vi "BRig_Host_v0,53.vi"() -> ()   [LabVIEW 2014]
uses:
  <vilib>/WebDAVClient/Advanced/SessionHandle.ctl
  BRig_Host__global__stopHost.vi
  <vilib>/Utility/file.llb/Write To Spreadsheet File (DBL).vi
  <vilib>/WebDAVClient/NI_WebDAV.lvlib
panel:
  out "FreeReward_c_R":u16
  out "FreeReward_c_L":u16
  out "BTPR_avg_R":dbl
  out "T2R_avg_R":dbl
  out "BTPR_avg_L":dbl
  out "T2R_avg_L":dbl
  out "BTPR_cur":u16
  out "T2R_cur":u16
  out "nReward":u16 caption="# Rewards in Current Block"
  out "BUR_target":u16 caption="Target Trials Per Block"
  out "nTrial":u16
  out "nReward_Right":u16 caption="# Rewards Total (Right)"
  out "nReward_Left":u16 caption="# Rewards Total (Left)"
  out "nReward_cur":u16 caption="# Rewards in Current Block"
  out "TpB_target":u16 caption="Target Trials Per Block"
  out "iBlock":u16 caption="Current Block"
  out "iTrial":u16 caption="Current Trial"
  out "DAB_nRewards_ProbLow_percent":u16 caption="# Rewards Total (Right)"
  out "DAB_nRewards_ProbHigh_percent":u16 caption="# Rewards Total (Left)"
  out "DAB_nRewards_ProbLow":u16 caption="# Rewards Total (Right)"
  out "DAB_nRewards_ProbHigh":u16 caption="# Rewards Total (Left)"
  out "DAB_nRewards_total":u16 caption="# Rewards in Current Block"
  out "DAB_nTrial":u16
  out "DAB_nRewards_Right":u16 caption="# Rewards Total (Right)"
  out "DAB_nRewards_Left":u16 caption="# Rewards Total (Left)"
  out "writeError":bool
  out "error IO":errorcluster
  out "error_loopP_loadSettings":errorcluster caption="error out"
  out "testCmdList":u16[][](array[numeric])
  in  "ClosedLoop":bool
  in  "module":string=" module1 "
  in  "input_updateTrial_subsequent":u16
  in  "input_updateTrial_first":u16
  in  "input_forceUpdate":bool
  in  "ClosedLoop":u16[](array[numeric])
  in  "testNewLaserSettings":bool
  in  "LoadSettings":bool
  in  "DisplayNumber":u16
  out "XY Graph":cluster{u16[], u16[]}[](graph)
  in  "threshold_2":u16=600
  in  "threshold_1":u16=300
  in  "Port (F=A/B, T=C)":bool
  out "I_ExpRun":bool
  out "TCP_connection":bool
  in  "stopHost":bool
  # "# Trials Displayed\n( 0 = all )"
  # "Selection\nTime Thresholds"
  # "Dual Armed Bandit"
  # "Standard or 2 Cues"
  # "Total"
  # "# Rewards"
  # "# Trials"
  # "Block Target"
  # "# Blocks"
  # "# Trials"
  # "# Rewards"
  # "Left           Right"
  # "Bad Trials\nPost Reward"
  # "Trials 2 Reward"
  # "Block"
  # "# Selections"
  # "# Trials"
  # "# Rewards"
  # "Current\nBlock"
  # "High Prob    Low Prob"
  # "avg L"
  # "Total"
  # "# Rewards"
  # "# Trials"
  # "avg R"
  # "% Selections"
  # "High Prob    Low Prob"
  # "FreeRewards"
  # "Left           Right"
  # "Port Switch\nToggle TRUE if debugging"
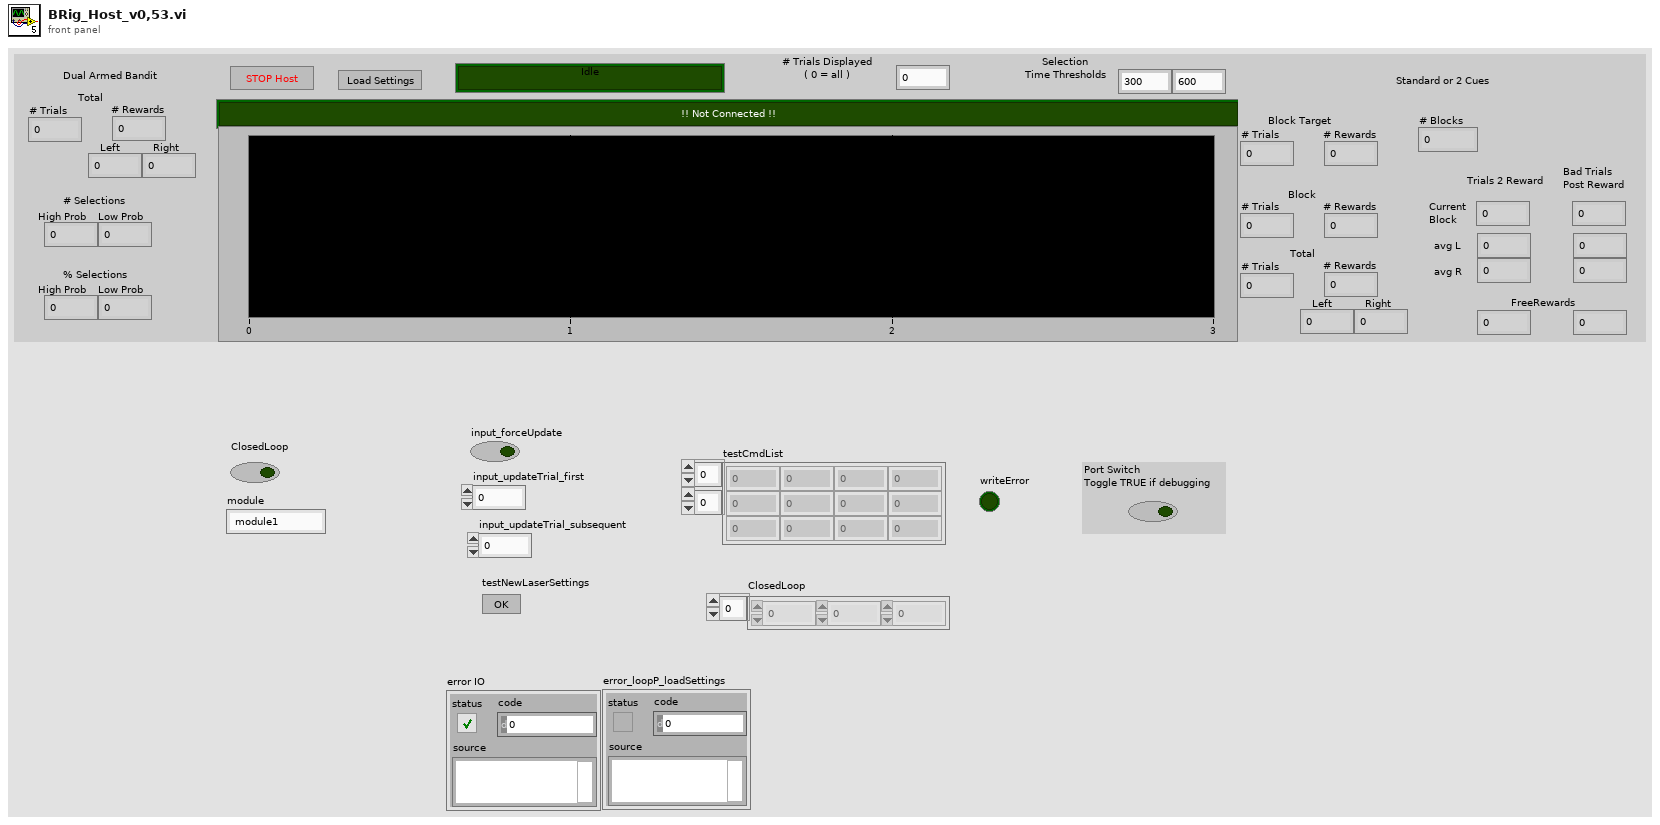
[diagram p1: front panel]
types:
  T1 = typedef "NI_WebDAV.lvlib/SessionHandle.ctl" = refnum<k1>
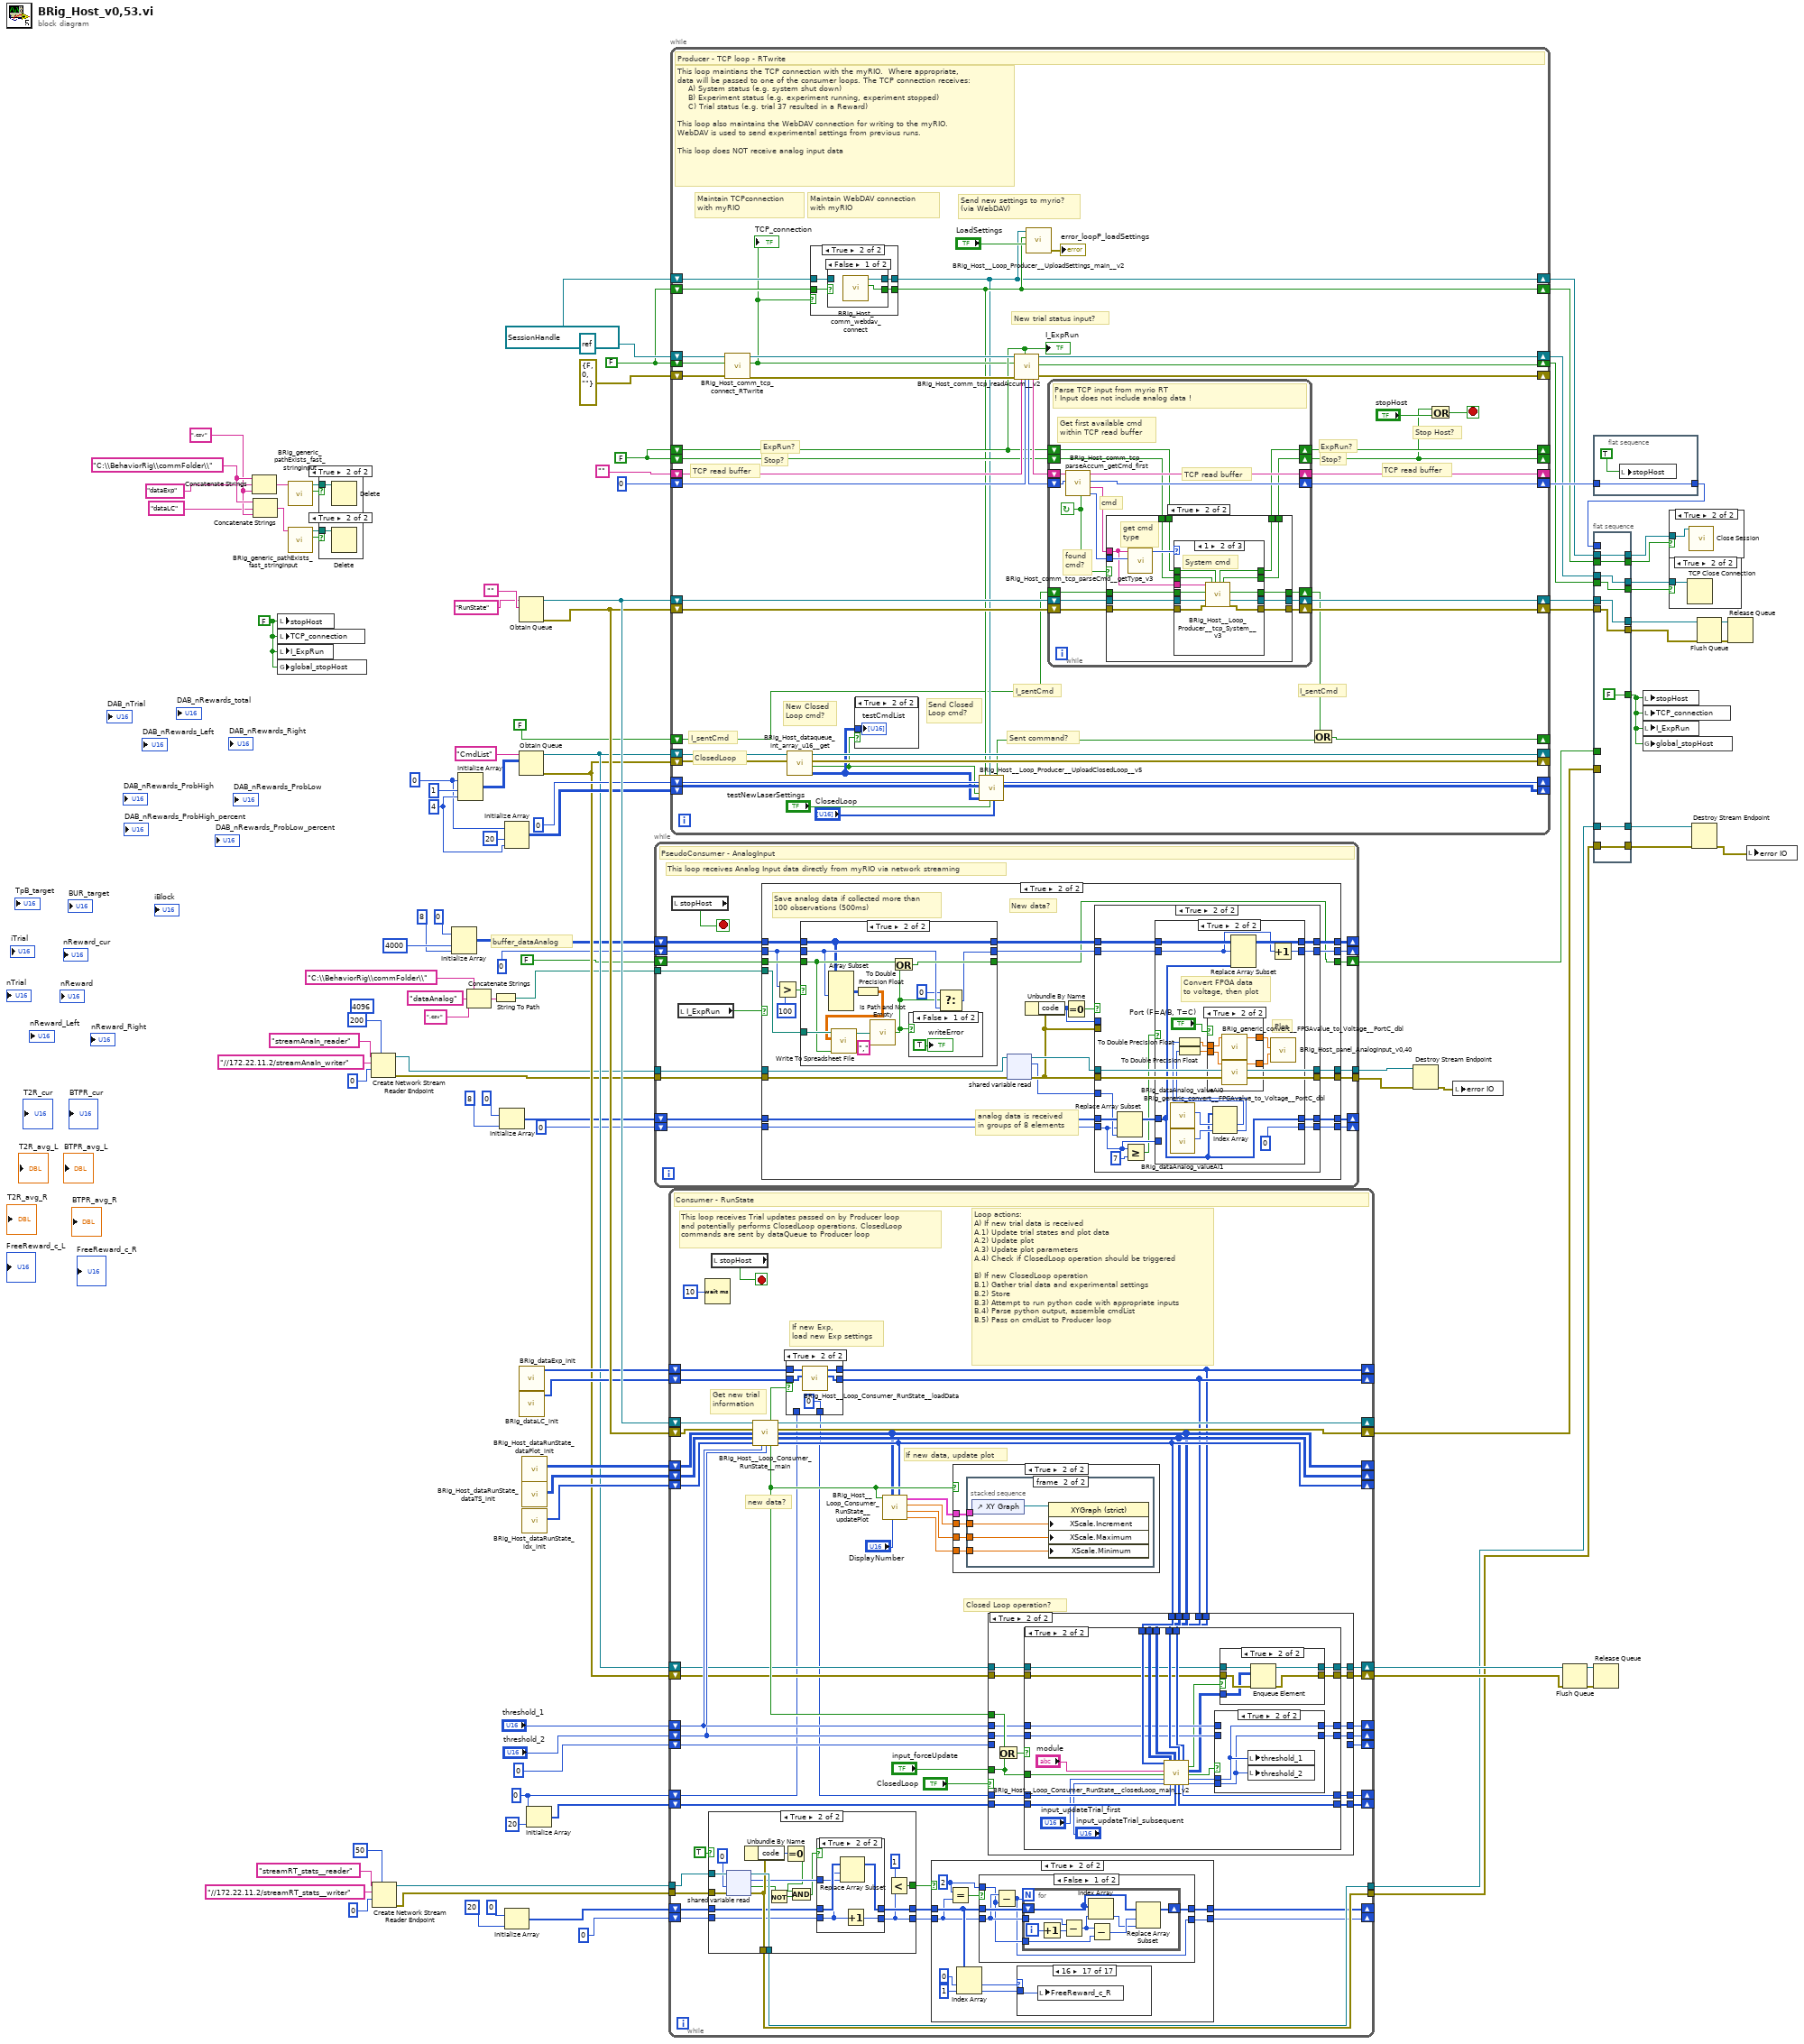
[diagram p0: block diagram]
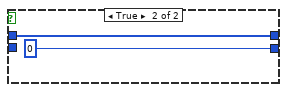
[diagram p9: hidden frame]
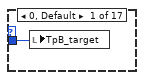
[diagram p10: hidden frame]
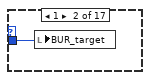
[diagram p11: hidden frame]
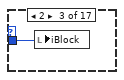
[diagram p12: hidden frame]
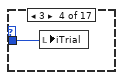
[diagram p13: hidden frame]
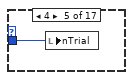
[diagram p14: hidden frame]
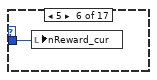
[diagram p15: hidden frame]
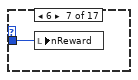
[diagram p16: hidden frame]
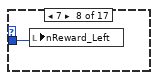
[diagram p17: hidden frame]
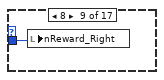
[diagram p18: hidden frame]
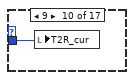
[diagram p19: hidden frame]
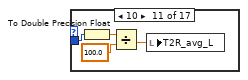
[diagram p20: hidden frame]
diagram:
  (unwired) 4096 ("reader buffer size")
  w41 = u16 0 ("element")
  w42 = 4 ("dimension size")
  w58 = u16 0
  w70 = ".csv" ("string")
  w71 = "C:\\BehaviorRig\\commFolder\\"
  w83 = T1 refnum items=["Session NI_WebDAV"] ("session handle")
  w101 = FALSE ("stopHost")
  w102 = FALSE
  w84 = FALSE
  # "buffer_dataAnalog"
  n1 = Concatenate Strings(w71, "dataExp" ("string"), w70) -> (w65:string)
  n2 = Concatenate Strings(w71, "dataLC" ("string"), w70) -> (w62:string)
  n3 = local write "stopHost"(w101) -> ()
  n4 = local write "TCP_connection"(w101) -> ()
  n5 = local write "I_ExpRun"(w101) -> ()
  n6 = global write "BRig_Host__global__stopHost.vi" "global_stopHost"(w101) -> ()
  n7 = call "BRig_generic_pathExists_fast_stringInput.vi"("input_filePath"=w65) -> ("output_Iexist"=w67:bool, "output_filePath"=w66:path)  [unwired: 8 in, 1 out]
  n8 = call "BRig_generic_pathExists_fast_stringInput.vi"("input_filePath"=w62) -> ("output_Iexist"=w63:bool, "output_filePath"=w64:path)  [unwired: 8 in, 1 out]
  n9 = case shown="True" w67 {
    tunnel: w66 -> [_ w107]
    frame False {
    }
    frame True {
      n10 = Delete(path (use dialog)=w107) -> ()  [unwired: 4 in, 3 out]
    }
  }
  n11 = case shown="True" w63 {
    tunnel: w64 -> [_ w108]
    frame False {
    }
    frame True {
      n12 = Delete(path (use dialog)=w108) -> ()  [unwired: 4 in, 3 out]
    }
  }
  n13 = Create Network Stream Reader Endpoint(7:200 ("reader buffer size"), 9:u16 0 ("element"), 10:"//172.22.11.2/streamAnaIn_writer" ("writer url"), 11:"streamAnaIn_reader" ("reader name")) -> (0:w25:errorcluster, 3:w26:refnum<k21>)  [unwired: 3 in]
  n14 = Create Network Stream Reader Endpoint(7:50 ("reader buffer size"), 9:u16 0 ("element"), 10:"//172.22.11.2/streamRT_stats__writer" ("writer url"), 11:"streamRT_stats__reader" ("reader name")) -> (0:w11:errorcluster, 3:w12:refnum<k21>)  [unwired: 3 in]
  n15 = Initialize Array(u16 0 ("element"), 4000 ("dimension size"), 8 ("dimension size")) -> (w37:u16[][])
  n16 = Initialize Array(w41, 1 ("dimension size"), w42) -> (w53:u16[][])
  n17 = Concatenate Strings("C:\\BehaviorRig\\commFolder\\" ("string"), "dataAnalog" ("input_filename"), ".csv" ("string")) -> (w34:string)
  n18 = String To Path(string=w34) -> (path=w31:path)
  n19 = Initialize Array(u16 0 ("element"), 8 ("dimension size")) -> (w18:u16[])
  n20 = Initialize Array(w41, 20 ("dimension size"), w42) -> (w72:u16[][])
  n21 = Initialize Array(u16 0 ("element"), 20 ("dimension size")) -> (w8:u16[])
  n22 = Obtain Queue(name (unnamed)="RunState", element data type="") -> (queue out=w93:refnum<queue>, error out=w92:errorcluster)  [unwired: 3 in, 1 out]
  n23 = Obtain Queue(name (unnamed)="CmdList", element data type=w53) -> (queue out=w52:refnum<queue>, error out=w51:errorcluster)  [unwired: 3 in, 1 out]
  n24 = call "BRig_dataExp_init.vi"() -> ("output_dataExp"=w61:u16[])  [unwired: 11 in]
  n25 = call "BRig_dataLC_init.vi"() -> ("output_dataLC"=w60:u16[])  [unwired: 11 in]
  n26 = call "BRig_Host_dataRunState_dataPlot_init.vi"() -> ("output_dataPlot"=w89:u16[][])  [unwired: 11 in]
  n27 = call "BRig_Host_dataRunState_dataTS_init.vi"() -> ("output_dataTS"=w88:u16[][])  [unwired: 11 in]
  n28 = call "BRig_Host_dataRunState_idx_init.vi"() -> ("output_idx"=w87:i32[])  [unwired: 11 in]
  n29 = Initialize Array(w58, 20 ("dimension size")) -> (w56:u16[])
  n30 = while {
    shift-right: [w123] -> _
    shift-left: w37 -> [w125]
    shift-right: [w122] -> _
    shift-left: 0 -> [w124]
    tunnel: w31 -> [w121]
    shift-right: [w119] -> w29
    shift-left: FALSE -> [w120]
    tunnel: w26 -> [w117]
    tunnel: w25 -> [w116]
    tunnel: [w115] -> w23
    tunnel: [w114] -> w22
    shift-right: [w111] -> _
    shift-left: w18 -> [w113]
    shift-right: [w110] -> _
    shift-left: 0 ("element") -> [w112]
    stop <- w109 stop-if-true
    # "This loop receives Analog Input data directly from myRIO via network streaming"
    # "PseudoConsumer - AnalogInput"
    n31 = local read "stopHost"() -> (w109:bool)
    n32 = local read "I_ExpRun"() -> (w118:bool)
    n33 = case shown="True" w118 {
      tunnel: w125 -> [w132 w156]
      tunnel: w124 -> [_ w142]
      tunnel: [w132 w151] -> w123
      tunnel: [0 w149] -> w122
      tunnel: w121 -> [_ w154]
      tunnel: w120 -> [_ w155]
      tunnel: [FALSE w139] -> w119
      tunnel: w117 -> [w129 w148]
      tunnel: w116 -> [w128 w147]
      tunnel: [w129 w145] -> w115
      tunnel: [w128 w143] -> w114
      tunnel: w113 -> [w127 w137]
      tunnel: w112 -> [_ w136]
      tunnel: [w127 w135] -> w111
      tunnel: [0 ("element") w134] -> w110
      frame False {
        n34 = Wait (ms)(milliseconds to wait=u32 20) -> ()  [unwired: 1 out]
      }
      frame True {
        # "analog data is received\nin groups of 8 elements"
        # "New data?"
        # "Save analog data if collected more than\n100 observations (500ms)"
        n35 = Greater?(x=w142, y=100) -> (0:w157:bool)
        n36 = case shown="True" w157 {
          tunnel: w156 -> [w216 w219]
          tunnel: [w216 w219] -> w152
          tunnel: w142 -> [w215 w221]
          tunnel: w155 -> [w214 w223]
          tunnel: [w215 w220] -> w150
          tunnel: [w214 w222] -> w139
          tunnel: w154 -> [_ w228]
          frame False {
          }
          frame True {
            n37 = Array Subset(array=w219, length (row)=w221) -> (w227:u16[][])  [unwired: 3 in]
            n38 = To Double Precision Float(number=w227) -> (double precision float=w226:dbl[][])
            n39 = call-poly <vilib>:"Write To Spreadsheet File.vi"("delimiter (\\t)"="," ("delimiter (\\t)"), "append to file? (new file:F)"=w223, "2D data"=w226, "file path (dialog if empty)"=w228) -> ("new file path (Not A Path if cancelled)"=w224:path)  [unwired: 4 in]
            n40 = call <vilib>:"Is Path and Not Empty.vi"("path"=w224) -> ("Is Path and Not Empty?"=w217:bool)  [unwired: 4 in]
            n41 = Or(x=w223, y=w217) -> (x .or. y?=w222:bool)
            n42 = case shown="False" w217 {
              frame False {
                "writeError" <- TRUE ("writeError")
              }
              frame True {
              }
            }
            n43 = Select(t=0, s=w217, f=w221) -> (s? t:f=w220:i32)
          }
        }
        n44 = shared-variable-read(w148, w147) -> (w146:refnum<k21>, w144:errorcluster, w138:u16)  [unwired: 1 in, 1 out]
        n45 = Unbundle By Name(w144) -> ("code"=w140:i32)
        n46 = Equal To 0?(x=w140) -> (x = 0?=w153:bool)
        n47 = case shown="True" w153 {
          tunnel: w152 -> [w170 w185]
          tunnel: [w170 w184] -> w151
          tunnel: w150 -> [w169 w183]
          tunnel: [w169 w182] -> w149
          tunnel: w144 -> [w167 _]
          tunnel: w146 -> [w166 w181]
          tunnel: [w166 w181] -> w145
          tunnel: w144 -> [w165 w180]
          tunnel: [w165 w180] -> w143
          tunnel: w140 -> [w164 _]
          tunnel: w138 -> [_ w178]
          tunnel: w137 -> [w159 w179]
          tunnel: w136 -> [w158 w176]
          tunnel: [w159 w173] -> w135
          tunnel: [w158 w175] -> w134
          frame False {
            n48 = Equal?(x=-314100, y=w164) -> (x = y?=w162:bool)
            n49 = Equal?(x=-314220, y=w164) -> (x = y?=w161:bool)
            n50 = Or(x=w162, y=w161) -> (x .or. y?=w160:bool)
            n51 = case shown="False" w160 {
              tunnel: w167 -> [w171 _]
              frame False {
                "error IO" <- w171
              }
              frame True {
              }
            }
          }
          frame True {
            n52 = Replace Array Subset(array=w179, new element=w178, index=w176) -> (w174:u16[])
            n53 = Greater Or Equal?(x=w176, y=7) -> (x >= y?=w172:bool)
            n54 = case shown="True" w172 {
              tunnel: w185 -> [w190 w205]
              tunnel: [w190 w204] -> w184
              tunnel: w183 -> [w189 w203]
              tunnel: [w189 w202] -> w182
              tunnel: w176 -> [w188 _]
              tunnel: [w187 0 ("y")] -> w175
              tunnel: w174 -> [w186 w193]
              tunnel: [w186 w193] -> w173
              frame False {
                n55 = Increment(x=w188) -> (x+1=w187:i32)
              }
              frame True {
                # "Convert FPGA data\nto voltage, then plot"
                # "Plot"
                n56 = call "BRig_dataAnalog_valueAI0.vi"() -> ("output_valueAI0"=w195:i32)  [unwired: 11 in]
                n57 = call "BRig_dataAnalog_valueAI1.vi"() -> ("output_valueAI1"=w196:i32)  [unwired: 11 in]
                n58 = Index Array(array=w193, index #1=w195, index #2=w196) -> (element #1=w192:u16, element #2=w191:u16)
                n59 = To Double Precision Float(number=w192) -> (double precision float=w197:dbl)
                n60 = To Double Precision Float(number=w191) -> (double precision float=w198:dbl)
                n61 = case shown="True" "Port (F=A/B, T=C)" {
                  tunnel: w197 -> [w207 w213]
                  tunnel: w198 -> [w206 w212]
                  tunnel: [w209 w211] -> w200
                  tunnel: [w208 w210] -> w199
                  frame False {
                    n62 = call "BRig_generic_convert__FPGAvalue_to_Voltage__PortAorB_dbl.vi"("input_FPGAvalue_PortAorB"=w207) -> ("output_voltage"=w209:dbl)  [unwired: 10 in]
                    n63 = call "BRig_generic_convert__FPGAvalue_to_Voltage__PortAorB_dbl.vi"("input_FPGAvalue_PortAorB"=w206) -> ("output_voltage"=w208:dbl)  [unwired: 10 in]
                  }
                  frame True {
                    n64 = call "BRig_generic_convert__FPGAvalue_to_Voltage__PortC_dbl.vi"("input_FPGAvalue_PortC"=w213) -> ("output_voltage"=w211:dbl)  [unwired: 10 in]
                    n65 = call "BRig_generic_convert__FPGAvalue_to_Voltage__PortC_dbl.vi"("input_FPGAvalue_PortC"=w212) -> ("output_voltage"=w210:dbl)  [unwired: 10 in]
                  }
                }
                n66 = Replace Array Subset(array=w205, new element=w193, index (row)=w203) -> (w204:u16[][])  [unwired: 1 in]
                n67 = Increment(x=w203) -> (x+1=w202:i32)
                n68 = call "BRig_Host_panel_AnalogInput_v0,40.vi"("graph_ai1"=w199, "graph_ai0"=w200) -> ()  [unwired: 10 in]
              }
            }
          }
        }
      }
    }
  }
  n69 = while {
    shift-right: [w274] -> _
    shift-left: w93 -> [w275]
    shift-right: [w272] -> w46
    shift-left: w92 -> [w273]
    shift-right: [w255] -> _
    shift-left: w89 -> [w271]
    shift-right: [w256] -> _
    shift-left: w88 -> [w270]
    shift-right: [w257] -> _
    shift-left: w87 -> [w269]
    shift-right: [w265] -> _
    shift-left: "threshold_1" -> [w264]
    shift-right: [w263] -> _
    shift-left: "threshold_2" -> [w262]
    shift-right: [w253] -> _
    shift-left: w61 -> [w267]
    shift-right: [w254] -> _
    shift-left: w60 -> [w266]
    shift-right: [w247] -> _
    shift-left: w58 -> [w245]
    shift-right: [w259] -> _
    shift-left: u8 0 -> [w260]
    shift-right: [w246] -> _
    shift-left: w56 -> [w243]
    shift-right: [w250] -> w48
    shift-left: w52 -> [w252]
    shift-right: [w249] -> w47
    shift-left: w51 -> [w251]
    tunnel: w12 -> [w241]
    tunnel: w11 -> [w240]
    shift-right: [w232] -> _
    shift-left: w8 -> [w237]
    shift-right: [w231] -> _
    shift-left: 0 ("element") -> [w236]
    tunnel: [w239] -> w4
    tunnel: [w238] -> w3
    stop <- w242 stop-if-true
    # "Closed Loop operation?"
    # "Loop actions:\nA) If new trial data is received\nA.1) Update trial states and plot data\nA.2) Update plot\nA.3) Update plot parameters\nA.4) Check if ClosedLoop operation should be triggered\n\nB) If new ClosedLoop operation\nB.1) Gather trial data and experimental settings\nB.2) Store\nB.3) Attempt to run python code with appropriate inputs\nB.4) Parse python output, assemble cmdList\nB.5) Pass on cmdList to Producer loop"
    # "This loop receives Trial updates passed on by Producer loop\nand potentially performs ClosedLoop operations. ClosedLoop\ncommands are sent by dataQueue to Producer loop"
    # "If new data, update plot"
    # "If new Exp,\nload new Exp settings"
    # "new data?"
    # "Get new trial\ninformation"
    # "Consumer - RunState"
    n70 = Wait (ms)(milliseconds to wait=u32 10) -> ()  [unwired: 1 out]
    n71 = case shown="True" TRUE {
      selector: TRUE -> [w282 _]
      tunnel: w241 -> [w286 w302]
      tunnel: w240 -> [w285 w301]
      tunnel: [w286 w300] -> w239
      tunnel: [w285 w299] -> w238
      tunnel: w237 -> [w284 w297]
      tunnel: w236 -> [w283 w296]
      tunnel: [w282 w294] -> w235
      tunnel: [w284 w293] -> w234
      tunnel: [w283 w292] -> w233
      frame False {
      }
      frame True {
        n72 = shared-variable-read(w302, w301, 0 ("timeout ms (-1)")) -> (w300:refnum<k21>, w299:errorcluster, w290:bool, w298:u16)
        n73 = Unbundle By Name(w299) -> ("code"=w303:i32)
        n74 = Not(x=w290) -> (.not. x?=w289:bool)
        n75 = Equal To 0?(x=w303) -> (x = 0?=w288:bool)
        n76 = And(x=w288, y=w289) -> (x .and. y?=w287:bool)
        n77 = case shown="True" w287 {
          tunnel: w298 -> [_ w309]
          tunnel: w297 -> [w305 w310]
          tunnel: w296 -> [w304 w308]
          tunnel: [w305 w306] -> w293
          tunnel: [w304 w307] -> w292
          frame False {
          }
          frame True {
            n78 = Replace Array Subset(array=w310, new element=w309, index=w308) -> (w306:u16[])
            n79 = Increment(x=w308) -> (x+1=w307:i32)
          }
        }
        n80 = Less?(x=1, y=w292) -> (x < y?=w294:bool)
      }
    }
    n81 = local read "stopHost"() -> (w242:bool)
    n82 = call "BRig_Host__Loop_Consumer_RunState__main.vi"("input_hDataQueue"=w275, "input_errorDataQueue"=w273, "input_dataPlot"=w271, "input_dataTS"=w270, "input_idx"=w269, "threshold_1"=w264, "threshold_2"=w262) -> ("output_ExpStart"=w268:bool, "output_hDataQueue"=w274:refnum<queue>, "output_errorDataQueue"=w272:errorcluster, "output_dataPlot"=w255:u16[][], "output_dataTS"=w256:u16[][], "output_updatePlot"=w258:bool, "output_idx"=w257:i32[])  [unwired: 2 in]
    n83 = case shown="True" w268 {
      tunnel: w267 -> [w451 w453]
      tunnel: [w451 w456] -> w253
      tunnel: w266 -> [w450 w454]
      tunnel: [w450 w455] -> w254
      tunnel: w245 -> [w449 _]
      tunnel: [w449 u16 0] -> w244
      frame False {
      }
      frame True {
        n84 = call "BRig_Host__Loop_Consumer_RunState__loadData.vi"("input_dataLC"=w454, "input_dataExp"=w453) -> ("output_dataLC"=w455:u16[], "output_dataExp"=w456:u16[])  [unwired: 8 in]
      }
    }
    n85 = call "BRig_Host__Loop_Consumer_RunState__updatePlot.vi"("input_idx"=w257, "input_DisplayNumber"="DisplayNumber", "input_dataPlot"=w255, "input_updatePlot"=w258) -> ("output_X_min"=w278:dbl, "output_X_max"=w277:dbl, "output_X_inc"=w276:dbl, "XY Graph"=w279:cluster{u16[], u16[]}[])  [unwired: 4 in]
    n86 = case shown="True" w235 {
      tunnel: w234 -> [w312 w317]
      tunnel: w233 -> [w311 w315]
      tunnel: [w312 w316] -> w232
      tunnel: [w311 w314] -> w231
      frame False {
      }
      frame True {
        w313 = 2 ("x")
        n87 = Equal?(x=w313, y=w315) -> (x = y?=w318:bool)
        n88 = Index Array(array=w317, index #1=0 ("index"), index #2=1 ("index")) -> (element #1=w320:u16, element #2=w319:u16)
        n89 = case shown="False" w318 {
          tunnel: w317 -> [w327 w338]
          tunnel: [w323 w338] -> w316
          tunnel: w315 -> [w326 _]
          tunnel: [w324 0 ("index")] -> w314
          tunnel: w313 -> [w325 _]
          frame False {
            n90 = Subtract(x=w326, y=w325) -> (x-y=w324:i32)
            n91 = for {
              N: w324 -> [_]
              shift-right: [w328] -> w323
              shift-left: w327 -> [w331]
              tunnel: w326 -> [w334]
              tunnel: w325 -> [w333]
              i -> [w336]
              n92 = Increment(x=w336) -> (x+1=w335:i32)
              n93 = Subtract(x=w334, y=w335) -> (x-y=w332:i32)
              n94 = Index Array(array=w331, index=w332) -> (element=w329:u16)
              n95 = Subtract(x=w332, y=w333) -> (x-y=w330:i32)
              n96 = Replace Array Subset(array=w331, new element=w329, index=w330) -> (w328:u16[])
            }
          }
          frame True {
          }
        }
        n97 = case shown="16" w320 {
          tunnel: w319 -> [w339 w340 w341 w342 w343 w344 w345 w346 w347 w348 w352 w356 w357 w359 w363 w366 w367]
          frame 0, Default {
            n98 = local write "TpB_target"(w339) -> ()
          }
          frame 1 {
            n99 = local write "BUR_target"(w340) -> ()
          }
          frame 2 {
            n100 = local write "iBlock"(w341) -> ()
          }
          frame 3 {
            n101 = local write "iTrial"(w342) -> ()
          }
          frame 4 {
            n102 = local write "nTrial"(w343) -> ()
          }
          frame 5 {
            n103 = local write "nReward_cur"(w344) -> ()
          }
          frame 6 {
            n104 = local write "nReward"(w345) -> ()
          }
          frame 7 {
            n105 = local write "nReward_Left"(w346) -> ()
          }
          frame 8 {
            n106 = local write "nReward_Right"(w347) -> ()
          }
          frame 9 {
            n107 = local write "T2R_cur"(w348) -> ()
          }
          frame 10 {
            n108 = To Double Precision Float(number=w352) -> (double precision float=w351:dbl)
            n109 = Divide(x=w351, y=100.0) -> (x/y=w349:dbl)
            n110 = local write "T2R_avg_L"(w349) -> ()
          }
          frame 11 {
            n111 = To Double Precision Float(number=w356) -> (double precision float=w355:dbl)
            n112 = Divide(x=w355, y=100.0) -> (x/y=w353:dbl)
            n113 = local write "T2R_avg_R"(w353) -> ()
          }
          frame 12 {
            n114 = local write "BTPR_cur"(w357) -> ()
          }
          frame 13 {
            n115 = To Double Precision Float(number=w359) -> (double precision float=w361:dbl)
            n116 = Divide(x=w361, y=100.0) -> (x/y=w358:dbl)
            n117 = local write "BTPR_avg_L"(w358) -> ()
          }
          frame 14 {
            n118 = To Double Precision Float(number=w363) -> (double precision float=w364:dbl)
            n119 = Divide(x=w364, y=100.0) -> (x/y=w362:dbl)
            n120 = local write "BTPR_avg_R"(w362) -> ()
          }
          frame 15 {
            n121 = local write "FreeReward_c_L"(w366) -> ()
          }
          frame 16 {
            n122 = local write "FreeReward_c_R"(w367) -> ()
          }
        }
      }
    }
    n123 = case shown="True" w258 {
      tunnel: w279 -> [_ w460]
      tunnel: w278 -> [_ w459]
      tunnel: w277 -> [_ w458]
      tunnel: w276 -> [_ w457]
      frame False {
      }
      frame True {
        n124 = stacked-sequence {
          tunnel: w460 -> [w461 _]
          tunnel: w459 -> [_ w464]
          tunnel: w458 -> [_ w463]
          tunnel: w457 -> [_ w462]
          frame #0 {
            "XY Graph" <- w461
          }
          frame #1 {
            n125 = control-ref of="XY Graph"() -> (w465:refnum<vi>)
            n126 = property class="XYGraph (strict)"(reference=w465, "XScale.Increment"=w462, "XScale.Maximum"=w463, "XScale.Minimum"=w464) -> ()  [unwired: 1 in, 2 out]
          }
        }
      }
    }
    n127 = case shown="True" "ClosedLoop" {
      tunnel: [w375 w398] -> w265
      tunnel: w264 -> [w376 w399]
      tunnel: [w374 w396] -> w263
      tunnel: w262 -> [w377 w397]
      tunnel: w260 -> [w380 _]
      tunnel: [w373 _] -> w259
      tunnel: w244 -> [w371 w403]
      tunnel: [w371 w401] -> w247
      tunnel: w243 -> [w370 w402]
      tunnel: [w370 w400] -> w246
      tunnel: w258 -> [_ w405]
      tunnel: w257 -> [_ w395]
      tunnel: w256 -> [_ w394]
      tunnel: w255 -> [_ w393]
      tunnel: w254 -> [_ w392]
      tunnel: w253 -> [_ w391]
      tunnel: w252 -> [w369 w390]
      tunnel: w251 -> [w368 w389]
      tunnel: [w369 w388] -> w250
      tunnel: [w368 w387] -> w249
      tunnel: "input_forceUpdate" -> [_ w386]
      frame False {
        n128 = Increment(x=w380) -> (x+1=w372:u8)
        n129 = Less?(x=w372, y=u8 10) -> (x < y?=w378:bool)
        n130 = case shown="False" w378 {
          tunnel: w377 -> [_ w384]
          tunnel: w376 -> [_ w385]
          tunnel: [w382 w385] -> w375
          tunnel: [w381 w384] -> w374
          tunnel: [_ w383] -> w373
          tunnel: w372 -> [_ w383]
          frame False {
            n131 = local read "threshold_1"() -> (w382:u16)
            n132 = local read "threshold_2"() -> (w381:u16)
          }
          frame True {
          }
        }
      }
      frame True {
        n133 = Or(x=w405, y=w386) -> (x .or. y?=w404:bool)
        n134 = case shown="True" w404 {
          tunnel: w386 -> [_ w434]
          tunnel: w403 -> [w411 w437]
          tunnel: w402 -> [w410 w436]
          tunnel: [w411 w430] -> w401
          tunnel: [w410 w431] -> w400
          tunnel: w399 -> [w409 w424]
          tunnel: [w409 w420] -> w398
          tunnel: w397 -> [w408 w423]
          tunnel: [w408 w419] -> w396
          tunnel: w395 -> [_ w429]
          tunnel: w394 -> [_ w428]
          tunnel: w393 -> [_ w427]
          tunnel: w392 -> [_ w426]
          tunnel: w391 -> [_ w425]
          tunnel: w390 -> [w407 w417]
          tunnel: w389 -> [w406 w415]
          tunnel: [w407 w416] -> w388
          tunnel: [w406 w414] -> w387
          frame False {
          }
          frame True {
            n135 = call "BRig_Host__Loop_Consumer_RunState__closedLoop_main__v2.vi"("input_idx"=w429, "input_module"="module", "input_forceUpdate"=w434, "input_updateTrial_first"="input_updateTrial_first", "input_updateTrial_subsequent"="input_updateTrial_subsequent", "input_dataTS"=w428, "input_updateID"=w437, "input_dataPlot"=w427, "input_trialList"=w436, "input_dataLC"=w426, "input_dataExp"=w425) -> ("output_trialList"=w431:u16[], "output_updateID"=w430:u16, 15:"output_cmdList"=w412:bool, 16:"output_cmdList"=w413:u16[][], "output_thres"=w418:bool, "output_thres1"=w422:u16, "output_thres2"=w421:u16)  [unwired: 2 in]
            n136 = case shown="True" w418 {
              tunnel: w424 -> [w446 _]
              tunnel: w423 -> [w445 _]
              tunnel: w422 -> [_ w448]
              tunnel: w421 -> [_ w447]
              tunnel: [w446 w448] -> w420
              tunnel: [w445 w447] -> w419
              frame False {
              }
              frame True {
                n137 = local write "threshold_1"(w448) -> ()
                n138 = local write "threshold_2"(w447) -> ()
              }
            }
            n139 = case shown="True" w412 {
              tunnel: w417 -> [w439 w444]
              tunnel: [w439 w441] -> w416
              tunnel: w415 -> [w438 w443]
              tunnel: [w438 w440] -> w414
              tunnel: w413 -> [_ w442]
              frame False {
              }
              frame True {
                n140 = Enqueue Element(queue=w444, element=w442, error in (no error)=w443) -> (queue out=w441:refnum<queue>, error out=w440:errorcluster)  [unwired: 1 in, 1 out]
              }
            }
          }
        }
      }
    }
  }
  n141 = while {
    shift-right: [w492] -> w77
    shift-left: w84 -> [w512]
    shift-right: [w507] -> w78
    shift-left: refnum<k5> refnum ("output_hTCP") -> [w511]
    shift-right: [w506] -> _
    shift-left: errorcluster {"status"=FALSE, "code"=0, "source"=""} ("output_error") -> [w510]
    shift-right: [w501] -> _
    shift-left: "" ("input_strAccum") -> [w505]
    shift-right: [w500] -> w91
    shift-left: 0 ("input_count") -> [w504]
    shift-right: [w499] -> _
    shift-left: w102 -> [w477]
    shift-right: [w475] -> _
    shift-left: w102 -> [w497]
    shift-right: [w494] -> w97
    shift-left: w93 -> [w496]
    shift-right: [w493] -> w96
    shift-left: w92 -> [w495]
    shift-right: [w472] -> w82
    shift-left: w84 -> [w491]
    shift-right: [w471] -> w81
    shift-left: w83 -> [w490]
    shift-right: [w482] -> _
    shift-left: w72 -> [w483]
    shift-right: [w466] -> _
    shift-left: 0 -> [w484]
    shift-right: [w486] -> _
    shift-left: w52 -> [w488]
    shift-right: [w485] -> _
    shift-left: w51 -> [w487]
    shift-right: [w467] -> _
    shift-left: FALSE -> [w470]
    stop <- w474 stop-if-true
    # "ClosedLoop"
    # "TCP read buffer"
    # "TCP read buffer"
    # "I_sentCmd"
    # "Sent command?"
    # "I_sentCmd"
    # "I_sentCmd"
    # "Stop Host?"
    # "Send Closed\nLoop cmd?"
    # "New Closed\nLoop cmd?"
    # "New trial status input?"
    # "ExpRun?"
    # "Stop?"
    # "This loop maintians the TCP connection with the myRIO.  Where appropriate,\ndata will be passed to one of the consumer loops. The TCP connection receives:\n    A) System status (e.g. system shut down)\n    B) Experiment status (e.g. experiment running, experiment stopped)\n    C) Trial status (e.g. trial 37 resulted in a Reward)\n\nThis loop also maintains the WebDAV connection for writing to the myRIO.\nWebDAV is used to send experimental settings from previous runs.\n\nThis loop does NOT receive analog input data"
    # "Send new settings to myrio?\n(via WebDAV)"
    # "ExpRun?"
    # "Stop?"
    # "Maintain TCPconnection\nwith myRIO"
    # "Maintain WebDAV connection\nwith myRIO"
    # "Producer - TCP loop - RTwrite"
    n142 = call "BRig_Host_comm_tcp_connect_RTwrite.vi"("input_error"=w510, "input_connected"=w512, "input_hTCP"=w511) -> ("output_error"=w508:errorcluster, "output_connected"=w476:bool, "output_hTCP"=w509:refnum<k5>)  [unwired: 5 in, 1 out]
    "TCP_connection" <- w476
    n143 = call "BRig_Host_dataqueue_int_array_u16__get.vi"("input_erroDataQueue"=w487, "input_hDataQueue"=w488) -> (0:"output_data"=w479:u16[][], 1:"output_data"=w478:bool, "output_errorDataQueue"=w485:errorcluster, "output_hDataQueue"=w486:refnum<queue>)  [unwired: 6 in]
    n144 = case shown="True" w476 {
      tunnel: w491 -> [w517 w525]
      tunnel: [w516 w524] -> w472
      tunnel: w490 -> [w515 w523]
      tunnel: [w514 w522] -> w471
      frame False {
        n145 = case shown="True" w517 {
          selector: w517 -> [w519 _]
          tunnel: [w519 FALSE] -> w516
          tunnel: w515 -> [w518 w520]
          tunnel: [w518 _] -> w514
          frame False {
          }
          frame True {
            n146 = call <vilib>:"Close Session.vi"("session handle"=w520) -> ()  [unwired: 14 in, 1 out]
          }
        }
      }
      frame True {
        n147 = case shown="False" w525 {
          selector: w525 -> [_ w529]
          tunnel: [w526 w529] -> w524
          tunnel: w523 -> [_ w528]
          tunnel: [w527 w528] -> w522
          frame False {
            n148 = call "BRig_Host_comm_webdav_connect.vi"() -> ("output_Iconnected"=w526:bool, "output_hSession"=w527:T1)  [unwired: 9 in, 1 out]
          }
          frame True {
          }
        }
      }
    }
    n149 = case shown="True" w478 {
      tunnel: w479 -> [_ w513]
      frame False {
      }
      frame True {
        "testCmdList" <- w513
      }
    }
    n150 = call "BRig_Host__Loop_Producer__UploadClosedLoop__v5.vi"("input_arrayBuffer_length"=w484, "input_arrayBuffer"=w483, 4:"input_cmdList"=w478, 5:"input_cmdList"=w479, "input_webdav_status"=w472, "session handle"=w471, "testNewLaserSettings"="testNewLaserSettings", "input_array_LaserSettings"="ClosedLoop") -> ("Sent"=w468:bool, "output_arrayBuffer_length"=w466:i32, "output_arrayBuffer"=w482:u16[][])  [unwired: 9 in]
    n151 = call "BRig_Host_comm_tcp_readAccum__v2.vi"("input_handle_TCP"=w509, "input_connected"=w476, "input_error"=w508, "input_strAccum"=w505, "input_I_ExpRun"=w477, "input_count"=w504) -> ("output_count"=w502:i32, "output_strAccum"=w503:string, "output_handle_TCP"=w507:refnum<k5>, "output_connected"=w492:bool, "output_error"=w506:errorcluster)  [unwired: 9 in]
    n152 = call "BRig_Host__Loop_Producer__UploadSettings_main__v2.vi"("input_LoadSettings"="LoadSettings", "input_webdav_status"=w472, "session handle"=w471) -> ("error out"=→"error_loopP_loadSettings":errorcluster)  [unwired: 8 in]
    n153 = while {
      shift-right: [w543] -> w501
      shift-left: w503 -> [w546]
      shift-right: [w542] -> w500
      shift-left: w502 -> [w545]
      shift-right: [w538] -> w499
      shift-left: w477 -> [w539]
      shift-right: [w536] -> w475
      shift-left: w497 -> [w537]
      shift-right: [w532] -> w494
      shift-left: w496 -> [w535]
      shift-right: [w533] -> w493
      shift-left: w495 -> [w534]
      shift-right: [w530] -> w469
      shift-left: w470 -> [w531]
      stop <- w544 continue-if-true
      # "found\ncmd?"
      # "TCP read buffer"
      # "cmd"
      # "Get first available cmd\nwithin TCP read buffer"
      # "Parse TCP input from myrio RT\n! Input does not include analog data !"
      n154 = call "BRig_Host_comm_tcp_parseAccum_getCmd_first.vi"("input_count"=w545, "input_strAccum"=w546) -> ("output_countCmd"=w540:i32, "output_strCmd"=w541:string, "output_count"=w542:i32, "output_strAccum"=w543:string, "output_I_cmd"=w544:bool)  [unwired: 5 in]
      n155 = case shown="True" w544 {
        tunnel: w541 -> [_ w562]
        tunnel: w540 -> [_ w564]
        tunnel: w539 -> [w551 w557]
        tunnel: [w551 w555] -> w538
        tunnel: w537 -> [w550 w556]
        tunnel: [w550 w554] -> w536
        tunnel: w535 -> [w549 w561]
        tunnel: w534 -> [w548 w560]
        tunnel: [w548 w559] -> w533
        tunnel: [w549 w558] -> w532
        tunnel: w531 -> [w547 w553]
        tunnel: [w547 w552] -> w530
        frame False {
        }
        frame True {
          # "get cmd\ntype"
          n156 = call "BRig_Host_comm_tcp_parseCmd__getType_v3.vi"("input_strCmd"=w562, "input_countCmd"=w564) -> ("output_strType"=w563:u8)  [unwired: 17 in]
          n157 = case shown="1" w563 {
            tunnel: w562 -> [_ w576 w588]
            tunnel: w561 -> [w569 w579 w587]
            tunnel: w560 -> [w568 w580 w586]
            tunnel: [w568 w578 w585] -> w559
            tunnel: [w569 w577 w584] -> w558
            tunnel: w557 -> [w567 w575 w583]
            tunnel: w556 -> [w566 w574 w582]
            tunnel: [w567 w573 w583] -> w555
            tunnel: [w566 w572 w582] -> w554
            tunnel: w553 -> [w565 w571 w581]
            tunnel: [w565 w570 w581] -> w552
            frame 0, Default {
              # "unknown cmd"
            }
            frame 1 {
              # "System cmd"
              n158 = call "BRig_Host__Loop_Producer__tcp_System__v3.vi"("input_strCmd"=w576, "input_I_SentCmd"=w571, "input_hDataQueue"=w579, "input_error_dataqueue"=w580, "input_I_Stop"=w574, "input_I_ExpRun"=w575) -> ("output_I_ExpRun"=w573:bool, "output_I_Stop"=w572:bool, "output_I_sentCmd"=w570:bool, "output_hDataQueue"=w577:refnum<queue>, "output_error"=w578:errorcluster)  [unwired: 9 in]
            }
            frame 2 {
              # "Send to\nconsumer loop"
              # "Trial state cmd"
              n159 = Enqueue Element(queue=w587, element=w588, error in (no error)=w586) -> (queue out=w584:refnum<queue>, error out=w585:errorcluster)  [unwired: 1 in, 1 out]
            }
          }
        }
      }
    }
    n160 = Or(x=w469, y=w468) -> (x .or. y?=w467:bool)
    n161 = Or(x=w475, y="stopHost") -> (x .or. y?=w474:bool)
    "I_ExpRun" <- w477
  }
  n162 = Destroy Stream Endpoint(8:w22, 11:w23) -> (0:w1:errorcluster)
  n163 = local write "error IO"(w1) -> ()
  n164 = Flush Queue(queue=w48, error in (no error)=w47) -> (queue out=w50:refnum<queue>, error out=w49:errorcluster)  [unwired: 1 out]
  n165 = flat-sequence {
    tunnel: w91 -> [w590]
    tunnel: [w590] -> w90
    frame #0 {
      n166 = local write "stopHost"(TRUE ("global_stopHost")) -> ()
    }
  }
  n167 = flat-sequence {
    tunnel: [FALSE] -> w100
    tunnel: w97 -> [w598]
    tunnel: w96 -> [w597]
    tunnel: [w598] -> w95
    tunnel: [w597] -> w94
    tunnel: w90 -> [_]
    tunnel: w82 -> [w595]
    tunnel: w81 -> [w596]
    tunnel: [w596] -> w79
    tunnel: [w595] -> w80
    tunnel: w78 -> [w593]
    tunnel: w77 -> [w594]
    tunnel: [w594] -> w76
    tunnel: [w593] -> w75
    tunnel: w46 -> [_]
    tunnel: w29 -> [_]
    tunnel: [w591] -> w6
    tunnel: [w592] -> w5
    tunnel: w4 -> [w592]
    tunnel: w3 -> [w591]
    frame #0 {
    }
  }
  n168 = Release Queue(queue=w50, error in (no error)=w49) -> ()  [unwired: 1 in, 3 out]
  n169 = local write "stopHost"(w100) -> ()
  n170 = local write "TCP_connection"(w100) -> ()
  n171 = local write "I_ExpRun"(w100) -> ()
  n172 = global write "BRig_Host__global__stopHost.vi" "global_stopHost"(w100) -> ()
  n173 = case shown="True" w80 {
    tunnel: w79 -> [_ w600]
    frame False {
    }
    frame True {
      n174 = call <vilib>:"Close Session.vi"("session handle"=w600) -> ()  [unwired: 14 in, 1 out]
    }
  }
  n175 = case shown="True" w76 {
    tunnel: w75 -> [_ w601]
    frame False {
    }
    frame True {
      n176 = TCP Close Connection(connection ID=w601) -> ()  [unwired: 2 in, 2 out]
    }
  }
  n177 = Destroy Stream Endpoint(8:w6, 11:w5) -> (0:w2:errorcluster)
  n178 = Flush Queue(queue=w95, error in (no error)=w94) -> (queue out=w45:refnum<queue>, error out=w44:errorcluster)  [unwired: 1 out]
  n179 = Release Queue(queue=w45, error in (no error)=w44) -> ()  [unwired: 1 in, 3 out]
  n180 = local write "error IO"(w2) -> ()
